vi "Create Header GenInfo.vi"(0 "dT":dbl, 2 "Nb Channels":i32, 4 "Nb Samples":i32, 6 "Time Type":enum16{"Response", "Drive"}(ring)) -> (13 "First X General parameters":i32, 14 "Binary Header Info":u8[][](array[numeric]), 16 "Nb Groups":i32, 18 "Total Nb Samples":i32)   [LabVIEW 2022 SP3, in "RPC.lvclass"]
uses:
  RPC.lvclass
panel:
  out "Nb Channels":i32
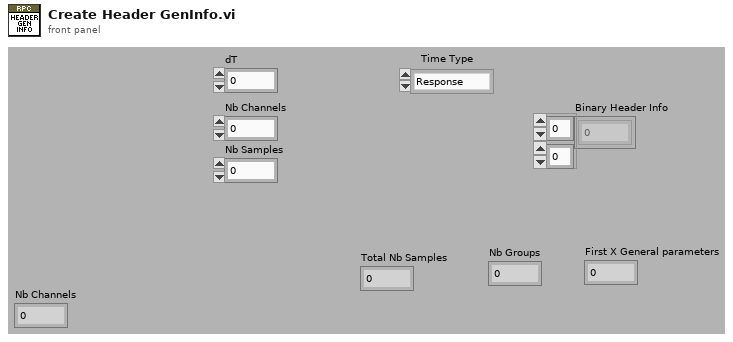
[diagram p1: front panel]
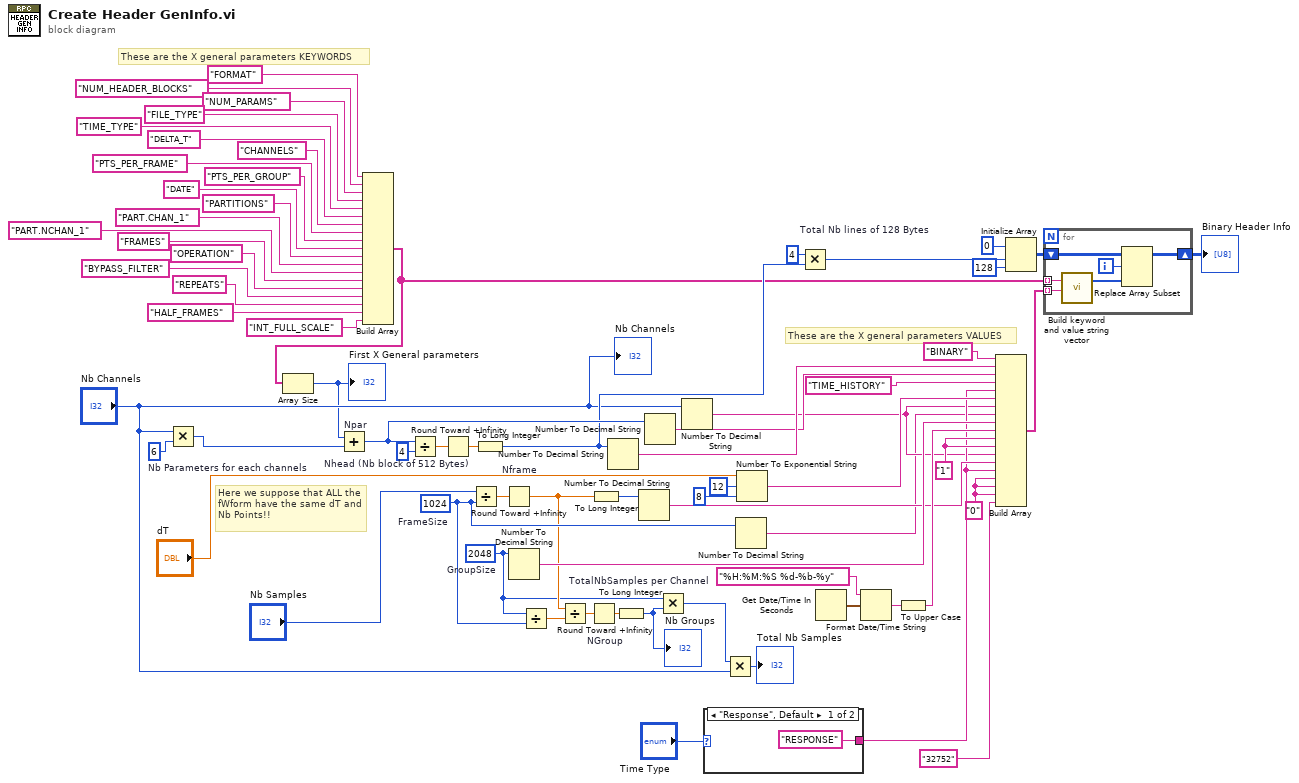
[diagram p0: block diagram]
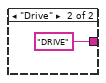
[diagram p2: hidden frame]
diagram:
  w28 = "1"
  w36 = "0"
  w69 = 6  # Nb Parameters for each channels
  w17 = 2048  # GroupSize
  w22 = 1024  # FrameSize
  # "These are the X general parameters VALUES"
  # "These are the X general parameters KEYWORDS"
  # "Here we suppose that ALL the fWform have the same dT and Nb Points!!"
  n1 = Multiply(x="Nb Channels", y=w69) -> (x*y=w44:i32)
  n2 = Build Array("FORMAT", "NUM_HEADER_BLOCKS", "NUM_PARAMS", "FILE_TYPE", "TIME_TYPE", "DELTA_T", "CHANNELS", "PTS_PER_FRAME", "PTS_PER_GROUP", "DATE", "PARTITIONS", "PART.CHAN_1", "PART.NCHAN_1", "FRAMES", "OPERATION", "BYPASS_FILTER", "REPEATS", "HALF_FRAMES", "INT_FULL_SCALE") -> (w8:string[])
  n3 = Array Size(array=w8) -> (size(s)=w7:i32)
  "First X General parameters" <- w7
  n4 = Add "Npar"(x=w7, y=w44) -> (x+y=w59:i32)
  n5 = Divide(x=w59, y=4) -> (x/y=w67:dbl)
  n6 = Round Toward +Infinity "Nhead (Nb block of 512 Bytes)"(x=w67) -> (ceil(x): smallest int >= x=w66:dbl)
  n7 = Divide(x="Nb Samples", y=w22) -> (x/y=w65:dbl)
  n8 = To Long Integer(number=w66) -> (32bit integer=w41:i32)
  n9 = Round Toward +Infinity "Nframe"(x=w65) -> (ceil(x): smallest int >= x=w21:dbl)
  n10 = Number To Decimal String(number=w17) -> (decimal integer string=w49:string)  [unwired: 1 out]
  n11 = Divide(x=w17, y=w22) -> (x/y=w20:dbl)
  n12 = Divide(x=w21, y=w20) -> (x/y=w18:dbl)
  n13 = Round Toward +Infinity "NGroup"(x=w18) -> (ceil(x): smallest int >= x=w19:dbl)
  n14 = To Long Integer(number=w21) -> (32bit integer=w47:i32)
  n15 = Number To Decimal String(number=w41) -> (decimal integer string=w61:string)  [unwired: 1 out]
  n16 = To Long Integer(number=w19) -> (32bit integer=w14:i32)
  "Nb Groups" <- w14
  n17 = Number To Decimal String(number=w47) -> (decimal integer string=w25:string)  [unwired: 1 out]
  n18 = Number To Decimal String(number=w59) -> (decimal integer string=w6:string)  [unwired: 1 out]
  n19 = Multiply "TotalNbSamples per Channel"(x=w17, y=w14) -> (x*y=w16:i32)
  n20 = Number To Decimal String(number="Nb Channels") -> (decimal integer string=w3:string)  [unwired: 1 out]
  n21 = case shown="\"Response\", Default" "Time Type" {
    tunnel: ["RESPONSE" "DRIVE"] -> w4
    frame "Response", Default {
    }
    frame "Drive" {
    }
  }
  n22 = Multiply ("TotalNbSamples")(x=w16, y="Nb Channels") -> (x*y=→"Total Nb Samples":i32)
  n23 = Number To Decimal String(number=w22) -> (decimal integer string=w2:string)  [unwired: 1 out]
  n24 = Number To Exponential String(number="dT", precision (6)=i16 8, 3:i16 12 ("width (-)")) -> (E-format string=w53:string)  [unwired: 1 out]
  n25 = Multiply "Total Nb lines of 128 Bytes"(x=4 ("y"), y=w41) -> (x*y=w39:i32)
  n26 = Get Date/Time In Seconds() -> (seconds since 1Jan1904=w34:timestamp)
  n27 = Format Date/Time String(time format string (%c)="%H:%M:%S %d-%b-%y", seconds (now)=w34) -> (date/time string=w33:string)  [unwired: 1 out]
  n28 = To Upper Case(1:w33) -> (0:w31:string)
  n29 = Build Array("BINARY", w61, w6, "TIME_HISTORY", w4, w53, w3, w2, w49, w31, w28, w28, w3, w25, w4, w36, w36, w36, "32752") -> (w46:string[])
  n30 = Initialize Array(u8 0 ("String"), w39, 128 ("dimension size")) -> (w42:u8[][])
  n31 = for {
    tunnel: w8 -> [w74] mode=indexing
    tunnel: w46 -> [w73] mode=indexing
    shift-right: [w75] -> w13
    shift-left: w42 -> [w77]
    i -> [w76]
    n32 = call "Build keyword and value string vector.vi"("Keywords"=w74, "Values"=w73) -> ("Keywords & Values in 128 Bytes vector"=w72:u8[])  [unwired: 17 in]
    n33 = Replace Array Subset(array=w77, new element=w72, index (row)=w76) -> (w75:u8[][])  [unwired: 1 in]
  }
  "Binary Header Info" <- w13
  "Nb Channels" <- "Nb Channels"
